vi "Constructor by Column.vi"(8 "error in (no error)":errorcluster, 9 "Field Configuration":refnum<class "Field Configuration.lvclass">, 10 "Basic Column":refnum<class "Column Interface.lvclass">, 11 "Ctrl Refnum Column in":refnum<class "Ctrl Refnum Column.lvclass">) -> (0 "error out":errorcluster, 3 "Ctrl Refnum Column out":refnum<class "Ctrl Refnum Column.lvclass">)   [LabVIEW 2020, in "Basic Fields.lvlib" / "Ctrl Refnum Column.lvclass"]
uses:
  Ctrl Refnum Column.lvclass
  Field Interfaces/Field Configuration Interface Class/Field Configuration.lvclass
  Column Interface/Column Interface Class/Column Interface.lvclass
  Basic Columns/Basic Columns/Column Class/Column Parent.lvclass
  Ctrl Refnum Column.lvclass/Ctrl Refnum Column.ctl
  Column Interface/Column Configuration Interface Class/Column Configuration.lvclass
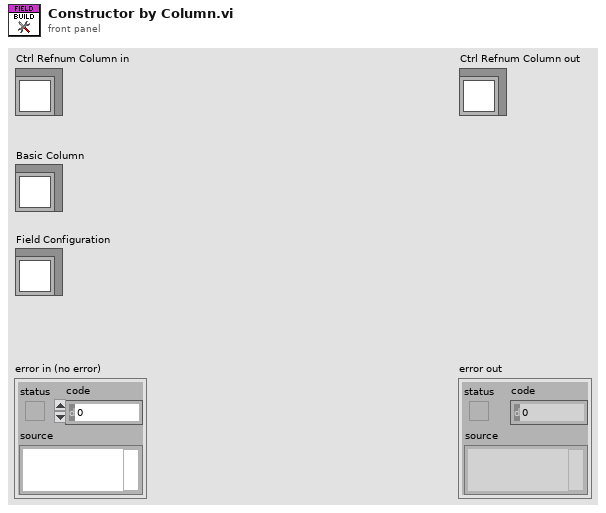
[diagram p1: front panel]
types:
  T1 = typedef "Database Interfaces.lvlib/Database data type.ctl" = enum16{"String", "Long (I32)", "Single (SGL)", "Double (DBL)", "Date/Time", "Binary"}
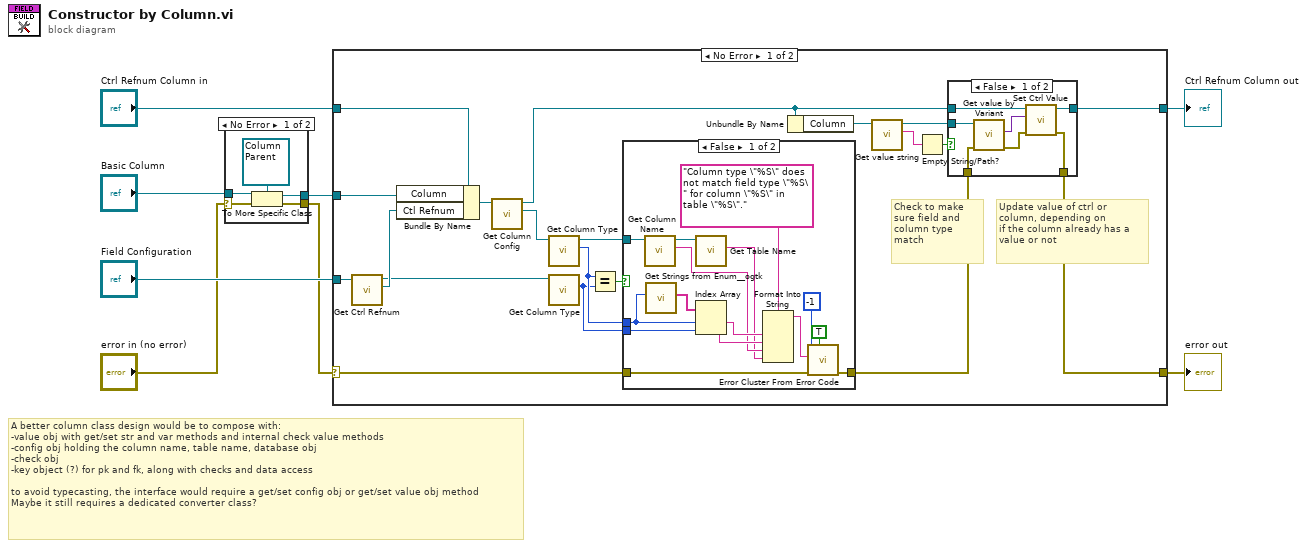
[diagram p0: block diagram]
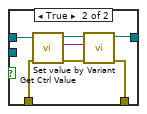
[diagram p3: hidden frame]
diagram:
  # "A better column class design would be to compose with:\n-value obj with get/set str and var methods and internal check value methods\n-config obj holding the column name, table name, database obj\n-check obj\n-key object (?) for pk and fk, along with checks and data access\n\nto avoid typecasting, the interface would require a get/set config obj or get/set value obj method\nMaybe it still requires a dedicated converter class?"
  n1 = case shown="No Error" "error in (no error)" {
    selector: "error in (no error)" -> [w10 w14]
    tunnel: "Basic Column" -> [w12 _]
    tunnel: [w11 _] -> w3
    tunnel: [w9 w14] -> w1
    frame No Error {
      n2 = To More Specific Class(target class=refnum<class "Column Parent.lvclass"> refnum ("Basic Columns.lvlib:Column Parent.lvclass"), reference=w12, error in=w10) -> (specific class reference=w11:refnum<class "Column Parent.lvclass">, error out=w9:errorcluster)
    }
    frame Error {
    }
  }
  n3 = case shown="No Error" w1 {
    selector: w1 -> [w26 w66]
    tunnel: [w15 w66] -> w8
    tunnel: [w17 w65] -> w6
    tunnel: "Ctrl Refnum Column in" -> [w34 w65]
    tunnel: "Field Configuration" -> [w33 _]
    tunnel: w3 -> [w31 _]
    frame No Error {
      # "Update value of ctrl or column, depending on\nif the column already has a value or not"
      # "Check to make sure field and column type match"
      n4 = call-dynamic "Get Ctrl Refnum.vi"("Field Configuration in"=w33) -> ("Ctl Refnum"=w32:refnum<vi>, "Field Configuration out"=w29:refnum<class "Field Configuration.lvclass">)  [unwired: 8 in, 1 out]
      n5 = Bundle By Name(cluster=w34, "Column"=w31, "Ctl Refnum"=w32) -> (w30:refnum<class "Ctrl Refnum Column.lvclass">)
      n6 = call-dynamic "Get Column Config.vi"("Ctrl Refnum Column in"=w30) -> ("Column Configuration"=w28:refnum<class "Column Configuration.lvclass">, "Ctrl Refnum Column out"=w18:refnum<class "Ctrl Refnum Column.lvclass">)  [unwired: 8 in, 1 out]
      n7 = call-dynamic "Get Column Type.vi"("Column Configuration in"=w28) -> ("Column Type"=w24:T1, "Column Configuration out"=w25:refnum<class "Column Configuration.lvclass">)  [unwired: 8 in, 1 out]
      n8 = call-dynamic "Get Column Type.vi"("Column Configuration in"=w29) -> ("Column Type"=w23:T1)  [unwired: 8 in, 2 out]
      n9 = Equal?(x=w24, y=w23) -> (x = y?=w27:bool)
      n10 = case shown="False" w27 {
        tunnel: w26 -> [w49 w64]
        tunnel: [w53 w64] -> w16
        tunnel: w25 -> [w63 _]
        tunnel: w24 -> [w59 _]
        tunnel: w23 -> [w60 _]
        frame False {
          n11 = call-dynamic "Get Column Name.vi"("Column Configuration in"=w63) -> ("Column Name"=w55:string, "Column Configuration out"=w62:refnum<class "Column Configuration.lvclass">)  [unwired: 8 in, 1 out]
          n12 = call <userlib>:"Get Strings from Enum__ogtk.vi"("Enum"=w59) -> ("Enum Strings"=w61:string[])  [unwired: 7 in, 3 out]
          n13 = call-dynamic "Get Table Name.vi"("Column Configuration in"=w62) -> ("Table Name"=w54:string)  [unwired: 8 in, 2 out]
          n14 = Index Array(array=w61, index #1=w59, index #2=w60) -> (element #1=w57:string, element #2=w56:string)
          n15 = Format Into String(format string="Column type \"%S\" does not match field type \"%S\" for column \"%S\" in table \"%S\".", w57, w56, w55, w54) -> (resulting string=w52:string)  [unwired: 2 in, 1 out]
          n16 = call <vilib>:"Error Cluster From Error Code.vi"("show call chain? (False)"=TRUE, "error in (no error)"=w49, "error message (\"\")"=w52, "error code (0)"=-1) -> ("error out"=w53:errorcluster)  [unwired: 5 in]
        }
        frame True {
        }
      }
      n17 = Unbundle By Name(w18) -> ("Column"=w21:refnum<class "Column Parent.lvclass">)
      n18 = call-dynamic "Get value string.vi"("Column in"=w21) -> ("Value"=w22:string, "Column out"=w19:refnum<class "Column Parent.lvclass">)  [unwired: 8 in, 1 out]
      n19 = Empty String/Path?(string/path=w22) -> (empty?=w20:bool)
      n20 = case shown="False" w20 {
        tunnel: w19 -> [w41 _]
        tunnel: w18 -> [w39 w48]
        tunnel: [w38 w45] -> w17
        tunnel: w16 -> [w37 w44]
        tunnel: [w35 w42] -> w15
        frame False {
          n21 = call-dynamic "Get value by Variant.vi"("error in (no error)"=w37, "Column Parent in"=w41) -> ("error out"=w36:errorcluster, "Variant"=w40:variant)  [unwired: 7 in, 1 out]
          n22 = call-dynamic "Set Ctrl Value.vi"("error in (no error)"=w36, "Variant"=w40, "Ctrl Refnum Column in"=w39) -> ("error out"=w35:errorcluster, "Ctrl Refnum Column out"=w38:refnum<class "Ctrl Refnum Column.lvclass">)  [unwired: 7 in]
        }
        frame True {
          n23 = call-dynamic "Get Ctrl Value.vi"("error in (no error)"=w44, "Ctrl Refnum Column in"=w48) -> ("error out"=w43:errorcluster, "Ctrl Value"=w46:variant, "Ctrl Refnum Column out"=w47:refnum<class "Ctrl Refnum Column.lvclass">)  [unwired: 7 in]
          n24 = call-dynamic "Set value by Variant.vi"("error in (no error)"=w43, "Variant"=w46, "Column in"=w47) -> ("error out"=w42:errorcluster, "Column out"=w45:refnum<class "Ctrl Refnum Column.lvclass">)  [unwired: 7 in]
        }
      }
    }
    frame Error {
    }
  }
  "error out" <- w8
  "Ctrl Refnum Column out" <- w6
